vi "Error Code Offset global.vi"() -> ()   [LabVIEW 2020]
doc: "A global variable that contains the <B>error code offset</B>s for..\n\n1. error codes returned from DLL function calls to the Andor MCD SDK (default 20000)\n\n2. error codes (in error clusters) returned from SubVI calls to the Andor MCD SDK for LabVIEW (default 5000)\n\nThe need to offset the error code from the DLL world to the LabVIEW world is due to the fact that LabVIEW has allocated most numbers for other kinds of errors. Third party software may use error codes in range 5000-9999, according to the documentation of the <B>General Error Handler.vi</B>."
panel:
  in  "ECO For LabVIEW":u32=5000
  in  "ECO For DLL":u32=20000
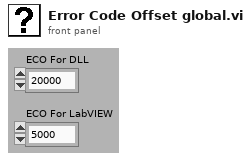
[diagram p1: front panel]
diagram:
